vi "initialize.vi"(8 "error in (no error)":errorcluster, 11 "name":string) -> (0 "error out":errorcluster, 3 "function return":i32)   [LabVIEW 2021, in "libad4.lvlib"]
doc: "LIBAD4 function: ad_open (const char_t *name);\n\nOpens a connection with the data acquisition system, using the passed `name` to identify the correct device. The `name` string is case-insensitive. This function returns a handle on success and -1 on error."
uses:
  <userlib>/libad4/libad4.lvlib
  <userlib>/libad4/libad4.dll
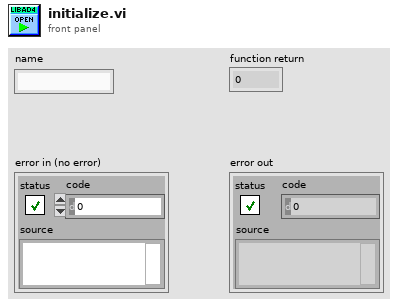
[diagram p1: front panel]
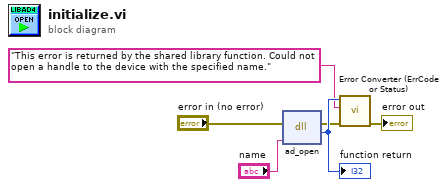
[diagram p0: block diagram]
diagram:
  n1 = dll-call lib="C:/Program Files/National Instruments/LabVIEW 2021/user.lib/libad4/libad4.*" fn="ad_open"(error in="error in (no error)", "name"="name") -> (error out=w3:errorcluster, w6:i32)  [unwired: 3 in, 1 out]
  "function return" <- w6
  n2 = call <userlib>:"Error Converter (ErrCode or Status).vi"("error in (no error)"=w3, "string"="This error is returned by the shared library function. Could not open a handle to the device with the specified name.", "error code"=w6) -> ("error out"=→"error out":errorcluster)  [unwired: 8 in]
